vi "ModulatorStepwise.vi"(8 "error in (no error)":errorcluster, 10 "wave":dbl[](array[numeric]) format="%0.2f", 11 "physical channels":tag="Dev2/ao0") -> (0 "error out":errorcluster, 3 "task out":refnum<k21>)   [LabVIEW 2011]
uses:
  <vilib>/DAQmx/write.llb/DAQmx Write (Analog Wfm 1Chan NSamp).vi
  <vilib>/DAQmx/create/channels.llb/DAQmx Create Channel (AO-Voltage-Basic).vi
  <vilib>/DAQmx/configure/timing.llb/DAQmx Timing (Sample Clock).vi
  <vilib>/DAQmx/miscellaneous.llb/DAQmx Fill In Error Info.vi
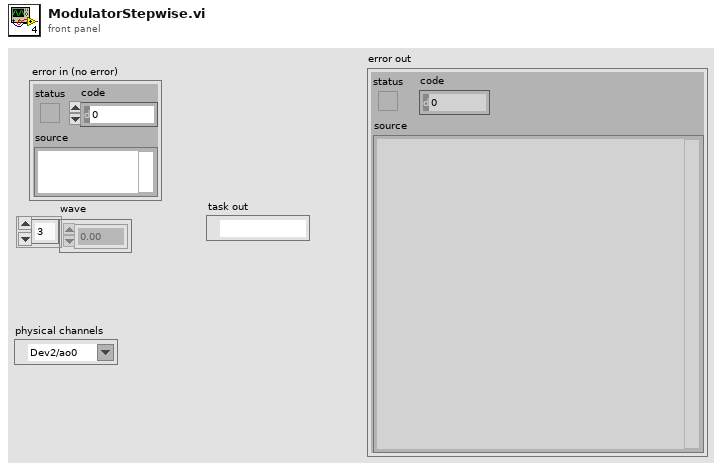
[diagram p1: front panel]
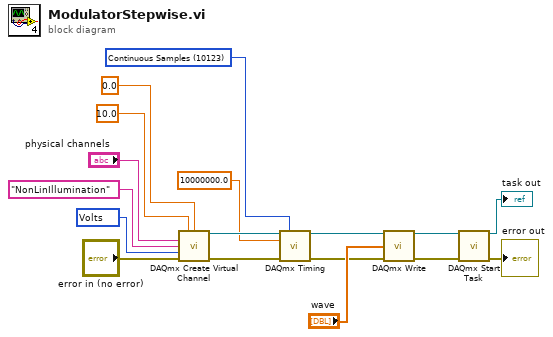
[diagram p0: block diagram]
diagram:
  w1 = 10123 items=["Finite Samples"=10178, "Continuous Samples"=10123, "Hardware Timed Single Point"=12522] ("sample mode")
  w13 = 10348 items=["Volts"=10348, "From Custom Scale"=10065] ("units")
  n1 = call-poly <vilib>:"DAQmx Create Virtual Channel.vi"("maximum value"=10.0, "minimum value"=0.0, "physical channels"="physical channels", "name to assign"="NonLinIllumination", "units"=w13, "error in"="error in (no error)") -> ("task out"=w4:refnum<k21>, "error out"=w6:errorcluster)  [unwired: 8 in]
  n2 = call-poly <vilib>:"DAQmx Timing.vi"("task/channels in"=w4, "sample mode"=w1, "rate"=10000000.0, "error in"=w6) -> ("task out"=w3:refnum<k21>, "error out"=w5:errorcluster)  [unwired: 10 in]
  n3 = call-poly <vilib>:"DAQmx Write.vi"("task/channels in"=w3, "data"="wave", "error in"=w5) -> ("task out"=w9:refnum<k21>, "error out"=w10:errorcluster)  [unwired: 10 in, 1 out]
  n4 = call <vilib>:"DAQmx Start Task.vi"("task/channels in"=w9, "error in"=w10) -> ("task out"=→"task out":refnum<k21>, "error out"=→"error out":errorcluster)  [unwired: 12 in]
